vi "Read Ini FIle bool.vi"(8 "error in (no error)":errorcluster, 9 "configuration file path":path, 10 "key":string[](array[string]), 11 "section":string[](array[string])) -> (0 "error out":errorcluster, 3 "CHMBtest":bool[](array[boolean]))   [LabVIEW 2023]
doc: "Read value (or values) from ini file and return double value (values)"
uses:
  <vilib>/Utility/config.llb/NI_LVConfig.lvlib
  <vilib>/Utility/config.llb/Read Key (String).vi
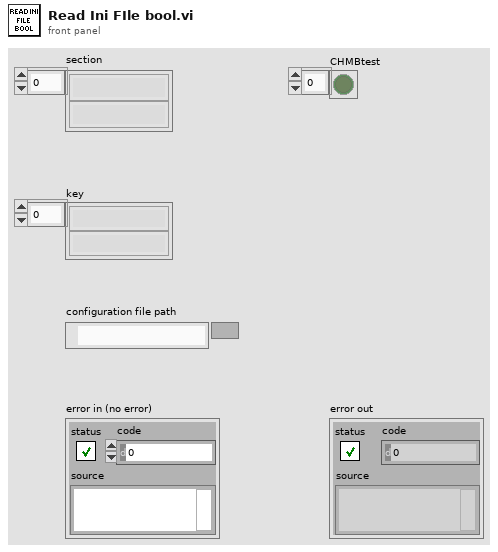
[diagram p1: front panel]
types:
  T1 = typedef "NI_LVConfig.lvlib/Config Data RefNum.ctl" = refnum<k1>
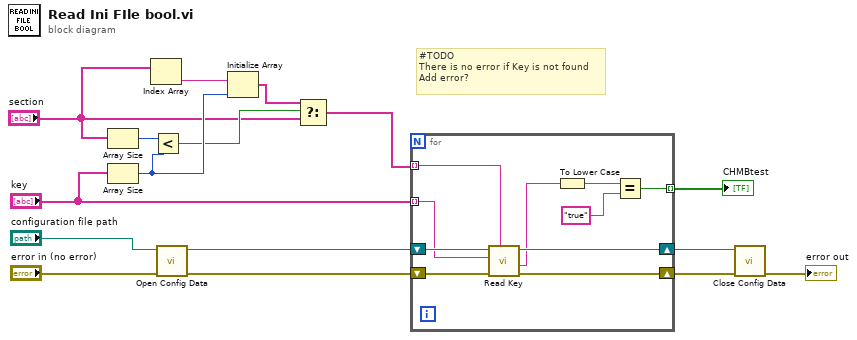
[diagram p0: block diagram]
diagram:
  # "#TODO\nThere is no error if Key is not found\nAdd error?"
  n1 = Array Size(array="section") -> (size(s)=w8:i32)
  n2 = Array Size(array="key") -> (size(s)=w6:i32)
  n3 = Index Array(array="section") -> (element=w7:string)  [unwired: 1 in]
  n4 = Less?(x=w8, y=w6) -> (x < y?=w5:bool)
  n5 = call <vilib>:"Open Config Data.vi"("error in (no error)"="error in (no error)", "configuration file path"="configuration file path") -> ("error out"=w14:errorcluster, "refnum"=w13:T1)  [unwired: 7 in, 1 out]
  n6 = Initialize Array(w7, w6) -> (w4:string[])
  n7 = Select(t=w4, s=w5, f="section") -> (s? t:f=w2:string[])
  n8 = for {
    tunnel: "key" -> [w24] mode=indexing
    tunnel: w2 -> [w23] mode=indexing
    shift-right: [w22] -> w12
    shift-left: w13 -> [w25]
    shift-right: [w21] -> w11
    shift-left: w14 -> [w26]
    tunnel: [w17] -> w1 mode=indexing
    n9 = call-poly <vilib>:"Read Key.vi"("section"=w23, "error in (no error)"=w26, "key"=w24, "refnum"=w25) -> ("error out"=w21:errorcluster, "value"=w19:string, "refnum out"=w22:T1)  [unwired: 4 in, 1 out]
    n10 = To Lower Case(string=w19) -> (all lower case string=w20:string)
    n11 = Equal?(x=w20, y="true") -> (x = y?=w17:bool)
  }
  "CHMBtest" <- w1
  n12 = call <vilib>:"Close Config Data.vi"("error in (no error)"=w11, "refnum"=w12) -> ("error out"=→"error out":errorcluster)  [unwired: 8 in, 1 out]
